vi "cw_6_2.vi"() -> ()   [LabVIEW 2022 SP3]
panel:
  out "Time Elapsed [ms] 4":dbl
  out "Time Elapsed [ms] 3":dbl
  out "Time Elapsed [ms] 2":dbl
  out "Time Elapsed [ms]":dbl
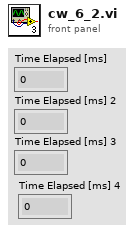
[diagram p1: front panel]
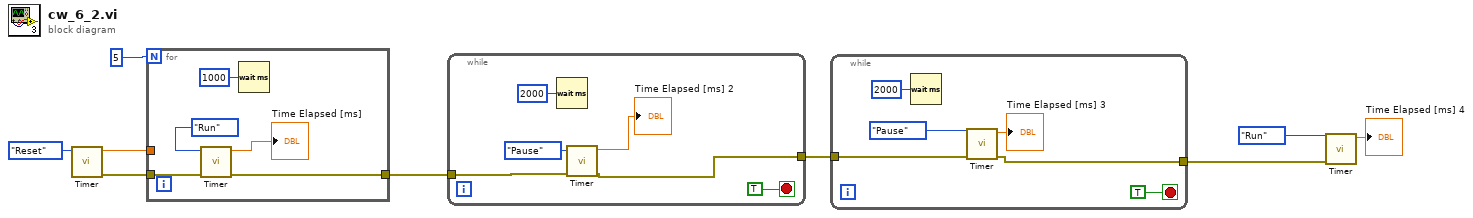
[diagram p0: block diagram]
diagram:
  n1 = call "Timer.vi"("Action"=enum16{"Pause", "Run", "Reset"}."Reset") -> ("error out"=w6:errorcluster, "Time Elapsed [ms]"=w7:dbl)  [unwired: 9 in]
  n2 = for {
    N: 5 -> [_]
    tunnel: w7 -> [_]
    tunnel: w6 -> [w12]
    tunnel: [w11] -> w5
    n3 = call "Timer.vi"("error in"=w12, "Action"=enum16{"Pause", "Run", "Reset"}."Run") -> ("error out"=w11:errorcluster, "Time Elapsed [ms]"=→"Time Elapsed [ms]":dbl)  [unwired: 8 in]
    n4 = Wait (ms)(milliseconds to wait=u32 1000) -> ()  [unwired: 1 out]
  }
  n5 = while {
    tunnel: w5 -> [w18]
    tunnel: [w16] -> w4
    stop <- TRUE stop-if-true
    n6 = Wait (ms)(milliseconds to wait=u32 2000) -> ()  [unwired: 1 out]
    n7 = call "Timer.vi"("error in"=w18, "Action"=enum16{"Pause", "Run", "Reset"}."Pause") -> ("error out"=w16:errorcluster, "Time Elapsed [ms]"=→"Time Elapsed [ms] 2":dbl)  [unwired: 8 in]
  }
  n8 = while {
    tunnel: w4 -> [w24]
    tunnel: [w22] -> w1
    stop <- TRUE stop-if-true
    n9 = Wait (ms)(milliseconds to wait=u32 2000) -> ()  [unwired: 1 out]
    n10 = call "Timer.vi"("error in"=w24, "Action"=enum16{"Pause", "Run", "Reset"}."Pause") -> ("error out"=w22:errorcluster, "Time Elapsed [ms]"=→"Time Elapsed [ms] 3":dbl)  [unwired: 8 in]
  }
  n11 = call "Timer.vi"("error in"=w1, "Action"=enum16{"Pause", "Run", "Reset"}."Run") -> ("Time Elapsed [ms]"=→"Time Elapsed [ms] 4":dbl)  [unwired: 8 in, 1 out]
